vi "#27_MAV_MSG_RAW_IMU.vi"(11 "mavlink_payload":u8[](array[numeric])) -> (3 "RAW_IMU":T1)   [LabVIEW 2023]
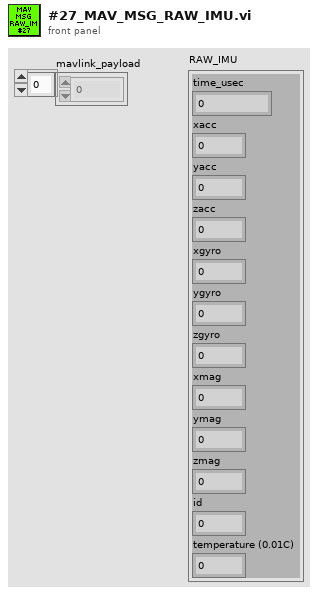
[diagram p1: front panel]
types:
  T1 = cluster{"time_usec":u64, "xacc":i16, "yacc":i16, "zacc":i16, "xgyro":i16, "ygyro":i16, "zgyro":i16, "xmag":i16, "ymag":i16, "zmag":i16, "id":u8, "temperature (0.01C)":i16}
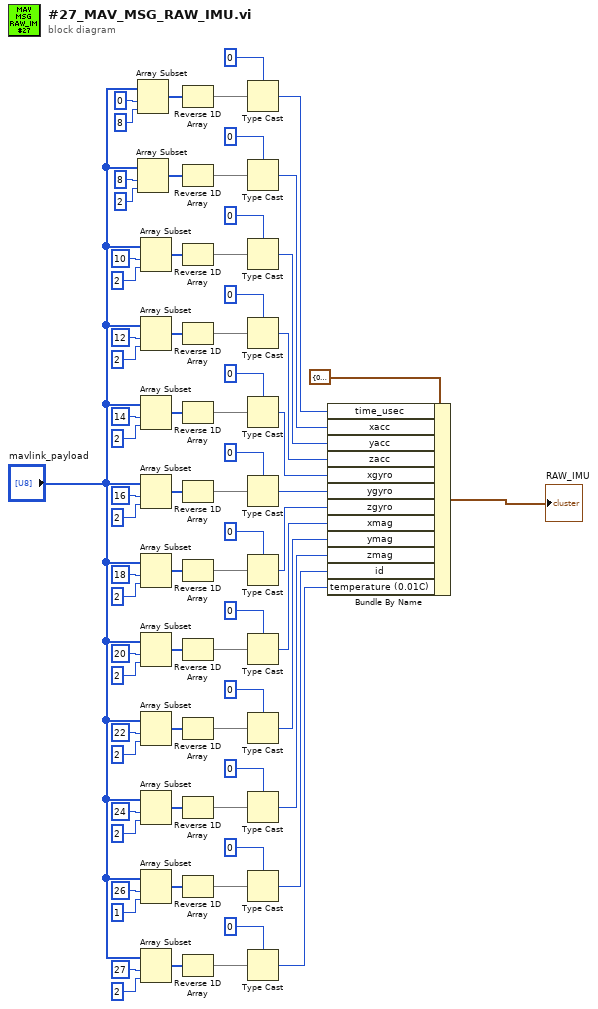
[diagram p0: block diagram]
diagram:
  n1 = Array Subset(array="mavlink_payload", index=0, length=8) -> (w73:u8[])
  n2 = Array Subset(array="mavlink_payload", index=8, length=2) -> (w65:u8[])
  n3 = Array Subset(array="mavlink_payload", index=10, length=2) -> (w59:u8[])
  n4 = Array Subset(array="mavlink_payload", index=12, length=2) -> (w53:u8[])
  n5 = Array Subset(array="mavlink_payload", index=14, length=2) -> (w47:u8[])
  n6 = Array Subset(array="mavlink_payload", index=16, length=2) -> (w41:u8[])
  n7 = Array Subset(array="mavlink_payload", index=18, length=2) -> (w35:u8[])
  n8 = Array Subset(array="mavlink_payload", index=20, length=2) -> (w29:u8[])
  n9 = Array Subset(array="mavlink_payload", index=22, length=2) -> (w23:u8[])
  n10 = Array Subset(array="mavlink_payload", index=24, length=2) -> (w17:u8[])
  n11 = Array Subset(array="mavlink_payload", index=26, length=1) -> (w11:u8[])
  n12 = Array Subset(array="mavlink_payload", index=27, length=2) -> (w5:u8[])
  n13 = Reverse 1D Array(array=w73) -> (reversed array=w72:u8[])
  n14 = Reverse 1D Array(array=w65) -> (reversed array=w64:u8[])
  n15 = Reverse 1D Array(array=w59) -> (reversed array=w58:u8[])
  n16 = Reverse 1D Array(array=w53) -> (reversed array=w52:u8[])
  n17 = Reverse 1D Array(array=w47) -> (reversed array=w46:u8[])
  n18 = Reverse 1D Array(array=w41) -> (reversed array=w40:u8[])
  n19 = Reverse 1D Array(array=w35) -> (reversed array=w34:u8[])
  n20 = Reverse 1D Array(array=w29) -> (reversed array=w28:u8[])
  n21 = Reverse 1D Array(array=w23) -> (reversed array=w22:u8[])
  n22 = Reverse 1D Array(array=w17) -> (reversed array=w16:u8[])
  n23 = Reverse 1D Array(array=w11) -> (reversed array=w10:u8[])
  n24 = Reverse 1D Array(array=w5) -> (reversed array=w4:u8[])
  n25 = Type Cast(type=u64 0 ("index"), x=w72) -> (*(type *) &x=w68:u64)
  n26 = Type Cast(type=i16 0 ("index"), x=w64) -> (*(type *) &x=w62:i16)
  n27 = Type Cast(type=i16 0 ("index"), x=w58) -> (*(type *) &x=w56:i16)
  n28 = Type Cast(type=i16 0 ("index"), x=w52) -> (*(type *) &x=w50:i16)
  n29 = Type Cast(type=i16 0 ("index"), x=w46) -> (*(type *) &x=w44:i16)
  n30 = Type Cast(type=i16 0 ("index"), x=w40) -> (*(type *) &x=w38:i16)
  n31 = Type Cast(type=i16 0 ("index"), x=w34) -> (*(type *) &x=w32:i16)
  n32 = Type Cast(type=i16 0 ("index"), x=w28) -> (*(type *) &x=w26:i16)
  n33 = Type Cast(type=i16 0 ("index"), x=w22) -> (*(type *) &x=w20:i16)
  n34 = Type Cast(type=i16 0 ("index"), x=w16) -> (*(type *) &x=w14:i16)
  n35 = Type Cast(type=u8 0 ("index"), x=w10) -> (*(type *) &x=w8:u8)
  n36 = Type Cast(type=i16 0 ("index"), x=w4) -> (*(type *) &x=w1:i16)
  n37 = Bundle By Name(cluster=T1 {"time_usec"=0, "xacc"=0, "yacc"=0, "zacc"=0, "xgyro"=0, "ygyro"=0, "zgyro"=0, "xmag"=0, "ymag"=0, "zmag"=0, "id"=0, "temperature (0.01C)"=0} ("RAW_IMU"), "time_usec"=w68, "xacc"=w62, "yacc"=w56, "zacc"=w50, "xgyro"=w44, "ygyro"=w38, "zgyro"=w32, "xmag"=w26, "ymag"=w20, "zmag"=w14, "id"=w8, "temperature (0.01C)"=w1) -> (→"RAW_IMU":T1)
